vi "Send status.vi"(8 "error in (no error)":errorcluster, 11 "Channel in":refnum<class "Channel.lvclass">) -> (0 "error out":errorcluster, 3 "Channel out":refnum<class "Channel.lvclass">)   [LabVIEW 2018, in "Channel.lvclass"]
uses:
  Channel.lvclass
  Channel.lvclass/Channel.ctl
  Header content/Header content.lvclass/Header content.ctl
  Server/Server.lvclass/Server.ctl
  Simulated_CCD_Camera/Simulated Camera.lvclass/Simulated Camera.ctl
  Server/Server.lvclass
  RxTx/CCS_RxTx.lvclass
  Simulated_CCD_Camera/Simulated Camera.lvclass
  Header content/Header content.lvclass
panel:
  in  "Prev SET parameters":T1
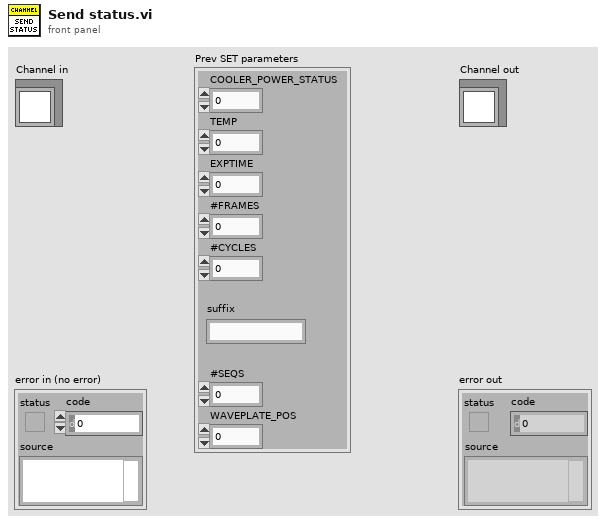
[diagram p1: front panel]
types:
  T1 = cluster{"COOLER_POWER_STATUS":u16, "TEMP":i32, "EXPTIME":dbl, "#FRAMES":u32, "#CYCLES":u32, "#SEQS":u32, "WAVEPLATE_POS":u16, "suffix":string}
  T2 = cluster{"CYCLES_DONE":u16, "LAST_IMAGE_NAME":string, "USED_DISK_SPACE":u16, "FRAMES_DONE":u16, "CCD_STATUS":string, "CURRENT_TEMPERATURE":i16, "TEMPERATURE_STATUS":string, "FRAME_EXPOSURE_TIME":sgl, "ERROR":bool, "SERIAL_NUMBER":u16, "ACQUIRING":bool, "IMAGE_INDEX":u32, "SEQS_DONE":u16}
  T3 = cluster{"PREAMP":u16, "READOUT_RATE":u16, "EM_GAIN":u16, "VERTICAL_SHIFT_SPEED":u16, "READ_MODE":u16, "FRAME_TRANSFER":bool, "VERTICAL_CLOCK_VOLTAGE":u16, "ACQUISITION_MODE":u16, "AD_CHANNEL":u16, "EM_MODE":u16, "SHUTTER_TTL":u16, "SHUTTER_OPENING_TIME":u16, "SHUTTER_CLOSING_TIME":u16, "SHUTTER_MODE":u16, "TRIGGER_MODE":u16, "VBIN":u16, "INITIAL_LINE":u16, "INITIAL_COLUMN":u16, "FINAL_LINE":u16, "FINAL_COLUMN":u16, "HBIN":u16}
  T4 = cluster{"COOLER_POWER_STATUS":u16, "TEMP":i32, "EXPTIME":dbl, "#FRAMES":u32, "#CYCLES":u32, "#SEQS":u32, "WAVEPLATE_POS":u16}
  T5 = cluster{"CCD status":string, "CCD configuration":string, "Acquisition configuration":string, "S4GUI JSON string":string}
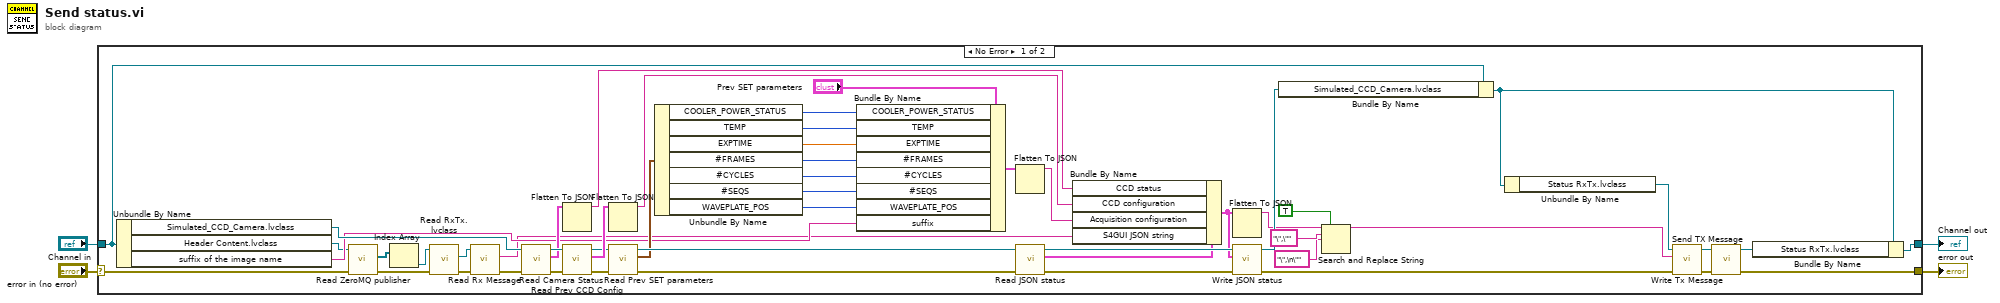
[diagram p0: block diagram]
diagram:
  n1 = case shown="No Error" "error in (no error)" {
    selector: "error in (no error)" -> [w12 w57]
    tunnel: [w50 w57] -> w3
    tunnel: [w49 w56] -> w1
    tunnel: "Channel in" -> [w48 w56]
    frame No Error {
      n2 = Unbundle By Name(w48) -> ("Simulated_CCD_Camera.lvclass"=w39:refnum<class "Simulated Camera.lvclass">, "Header Content.lvclass"=w13:refnum<class "Header content.lvclass">, "suffix of the image name"=w14:string)
      n3 = call "Read ZeroMQ publisher.vi"("error in (no error)"=w12, "Header content in"=w13) -> ("error out"=w8:errorcluster, "ZeroMQ publisher"=w11:refnum<class "Server.lvclass">[])  [unwired: 7 in, 1 out]
      n4 = Index Array(array=w11) -> (element=w9:refnum<class "Server.lvclass">)  [unwired: 1 in]
      n5 = call "Read RxTx.lvclass.vi"("error in (no error)"=w8, "Server in"=w9) -> ("error out"=w7:errorcluster, "RxTx.lvclass"=w10:refnum<class "CCS_RxTx.lvclass">)  [unwired: 7 in, 1 out]
      n6 = call "Read Rx Message.vi"("error in (no error)"=w7, "RxTx in"=w10) -> ("error out"=w6:errorcluster, "Rx Message"=w5:string)  [unwired: 7 in, 1 out]
      n7 = call "Read Camera Status.vi"("error in (no error)"=w6, "CCDCamera in"=w39) -> ("error out"=w38:errorcluster, "Camera Status"=w36:T2, "CCDCamera out"=w40:refnum<class "Simulated Camera.lvclass">)  [unwired: 7 in]
      n8 = Flatten To JSON(anything=w36) -> (JSON string=w37:string)  [unwired: 2 in, 1 out]
      n9 = call-dynamic "Read Prev CCD Config.vi"("error in (no error)"=w38, "Simulated_CCD_Camera in"=w40) -> ("error out"=w34:errorcluster, "Prev CCD Config"=w44:T3, "Simulated_CCD_Camera out"=w35:refnum<class "Simulated Camera.lvclass">)  [unwired: 7 in]
      n10 = Flatten To JSON(anything=w44) -> (JSON string=w45:string)  [unwired: 2 in, 1 out]
      n11 = call-dynamic "Read Prev SET parameters.vi"("error in (no error)"=w34, "Simulated_CCD_Camera in"=w35) -> ("error out"=w33:errorcluster, "Prev SET parameters"=w22:T4, "Simulated_CCD_Camera out"=w32:refnum<class "Simulated Camera.lvclass">)  [unwired: 7 in]
      n12 = Unbundle By Name(w22) -> ("COOLER_POWER_STATUS"=w21:u16, "TEMP"=w20:i32, "EXPTIME"=w19:dbl, "#FRAMES"=w18:u32, "#CYCLES"=w17:u32, "#SEQS"=w16:u32, "WAVEPLATE_POS"=w15:u16)
      n13 = Bundle By Name(cluster="Prev SET parameters", "COOLER_POWER_STATUS"=w21, "TEMP"=w20, "EXPTIME"=w19, "#FRAMES"=w18, "#CYCLES"=w17, "#SEQS"=w16, "WAVEPLATE_POS"=w15, "suffix"=w14) -> (w23:T1)
      n14 = Flatten To JSON(anything=w23) -> (JSON string=w31:string)  [unwired: 2 in, 1 out]
      n15 = call "Read JSON status.vi"("error in (no error)"=w33, "Simulated_CCD_Camera in"=w32) -> ("error out"=w46:errorcluster, "JSON status"=w26:T5, "Simulated_CCD_Camera out"=w47:refnum<class "Simulated Camera.lvclass">)  [unwired: 7 in]
      n16 = Bundle By Name(cluster=w26, "CCD status"=w37, "CCD configuration"=w45, "Acquisition configuration"=w31, "S4GUI JSON string"=w5) -> (w41:T5)
      n17 = Flatten To JSON(anything=w41) -> (JSON string=w30:string)  [unwired: 2 in, 1 out]
      n18 = call "Write JSON status.vi"("error in (no error)"=w46, "JSON status"=w41, "Simulated_CCD_Camera in"=w47) -> ("error out"=w42:errorcluster, "Simulated_CCD_Camera out"=w43:refnum<class "Simulated Camera.lvclass">)  [unwired: 7 in]
      n19 = Bundle By Name(cluster=w48, "Simulated_CCD_Camera.lvclass"=w43) -> (w55:refnum<class "Channel.lvclass">)
      n20 = Search and Replace String(replace all?=TRUE ("replace all? (F)"), input string=w30, search string="\",\"", replace string="\",\n\"" ("search string")) -> (result string=w25:string)  [unwired: 4 in, 3 out]
      n21 = Unbundle By Name(w55) -> ("Status RxTx.lvclass"=w51:refnum<class "CCS_RxTx.lvclass">)
      n22 = call "Write Tx Message.vi"("error in (no error)"=w42, "Tx Message"=w25, "RxTx in"=w51) -> ("error out"=w52:errorcluster, "RxTx out"=w54:refnum<class "CCS_RxTx.lvclass">)  [unwired: 7 in]
      n23 = call "Send TX Message.vi"("error in (no error)"=w52, "RxTx in"=w54) -> ("error out"=w50:errorcluster, "RxTx out"=w53:refnum<class "CCS_RxTx.lvclass">)  [unwired: 8 in]
      n24 = Bundle By Name(cluster=w55, "Status RxTx.lvclass"=w53) -> (w49:refnum<class "Channel.lvclass">)
    }
    frame Error {
    }
  }
  "error out" <- w3
  "Channel out" <- w1
